vi "TPG366_get_p.vi"(8 "error in (no error)":errorcluster, 10 "sensor_number":i32=1, 11 "connection ID":refnum<k5>) -> (0 "err_out":errorcluster, 2 "pressure":dbl caption="Torr", 3 "connection ID out":refnum<k5>, 4 "status":bool)   [LabVIEW 2019]
panel:
  out "comm":string
  out "bytes written":i32
  out "read_2":string
  out "read_1":string
  out "status_ack":bool
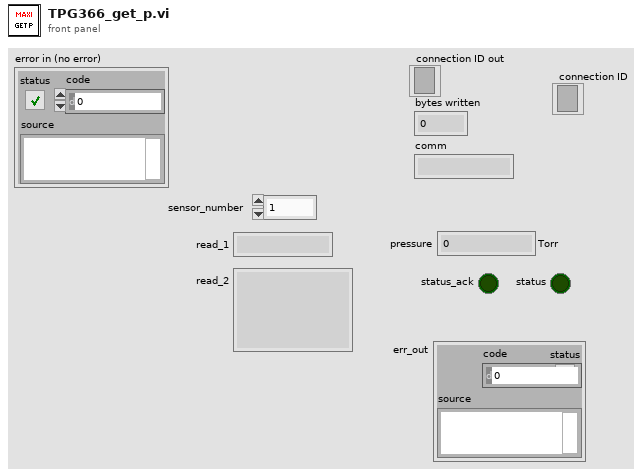
[diagram p1: front panel]
types:
  T1 = enum16{"Standard", "Buffered", "CRLF", "Immediate"}
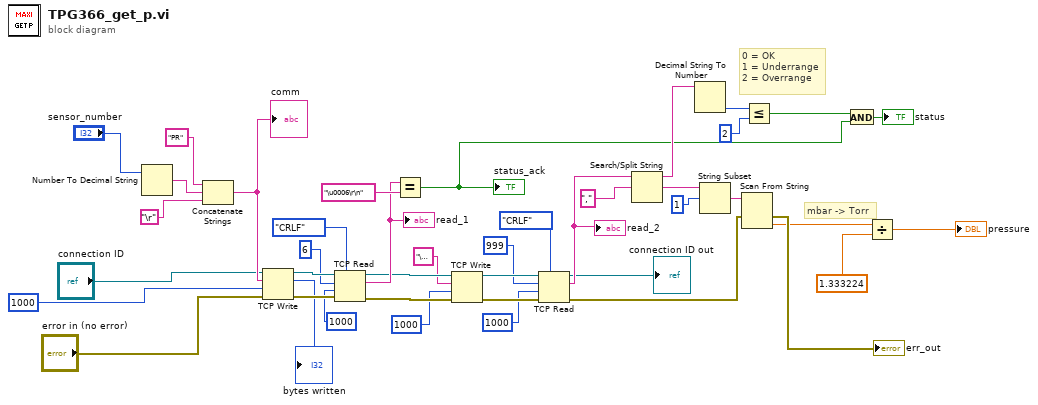
[diagram p0: block diagram]
diagram:
  # "0 = OK\n1 = Underrange\n2 = Overrange"
  # "mbar -> Torr"
  n1 = Number To Decimal String(number="sensor_number") -> (decimal integer string=w33:string)  [unwired: 1 in]
  n2 = Concatenate Strings("PR" ("string"), w33, "\r") -> (w24:string)
  "comm" <- w24
  n3 = TCP Write(connection ID="connection ID", data in=w24, error in (no error)="error in (no error)", 9:1000 ("timeout ms (25000)")) -> (connection ID out=w23:refnum<k5>, bytes written=→"bytes written":i32, error out=w22:errorcluster)
  n4 = TCP Read(connection ID=w23, bytes to read=6, error in (no error)=w22, 7:T1."CRLF" ("mode (standard)"), 9:1000 ("timeout ms (25000)")) -> (connection ID out=w16:refnum<k5>, data out=w17:string, error out=w15:errorcluster)
  "read_1" <- w17
  n5 = Equal?(x=w17, y="\u0006\r\n") -> (x = y?=w36:bool)
  "status_ack" <- w36
  n6 = TCP Write(connection ID=w16, data in="\u0005", error in (no error)=w15, 9:1000 ("timeout ms (25000)")) -> (connection ID out=w13:refnum<k5>, error out=w12:errorcluster)  [unwired: 1 out]
  n7 = TCP Read(connection ID=w13, bytes to read=999, error in (no error)=w12, 7:T1."CRLF" ("mode (standard)"), 9:1000 ("timeout ms (25000)")) -> (connection ID out=→"connection ID out":refnum<k5>, data out=w8:string, error out=w9:errorcluster)
  "read_2" <- w8
  n8 = Search/Split String(string=w8, search string/char (-)=",") -> (substring before match=w39:string, match + rest of string=w41:string)  [unwired: 1 in, 1 out]
  n9 = Decimal String To Number(string=w39) -> (number=w26:i32)  [unwired: 2 in, 1 out]
  n10 = String Subset(string=w41, offset (0)=1) -> (substring=w31:string)  [unwired: 1 in]
  n11 = Scan From String(input string=w31, error in=w9) -> (error out=→"err_out":errorcluster, output 1=w27:dbl)  [unwired: 3 in, 2 out]
  n12 = Less Or Equal?(x=w26, y=2) -> (x <= y?=w37:bool)
  n13 = And(x=w37, y=w36) -> (x .and. y?=→"status":bool)
  n14 = Divide(x=w27, y=1.333224) -> (x/y=→"pressure":dbl)
